vi "Read JSON from Stream.vi"(11 "Stream in":refnum<class "Stream.lvclass">) -> (0 "error out":errorcluster, 2 "Data":string)   [LabVIEW 2020, in "Stream-Simple-Msg.lvlib" / "Endpoint.lvclass"]
uses:
  Endpoint.lvclass
  <vilib>/IlluminatedG/lv-stream/stream/Stream.lvclass
  <vilib>/IlluminatedG/lv-web-crypto/lv-json/JSON/JSON Item Type.ctl
  <vilib>/IlluminatedG/lv-web-crypto/lv-json/JSON/JSON.lvlib
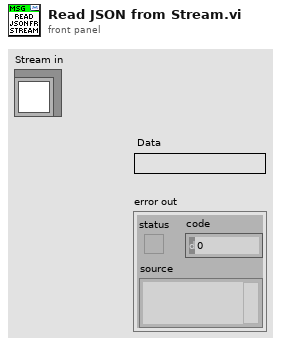
[diagram p1: front panel]
types:
  T1 = typedef "JSON.lvlib/JSON Item Type.ctl" = enum16{"unknown", "null", "Array", "Object", "String", "Number", "Boolean"}
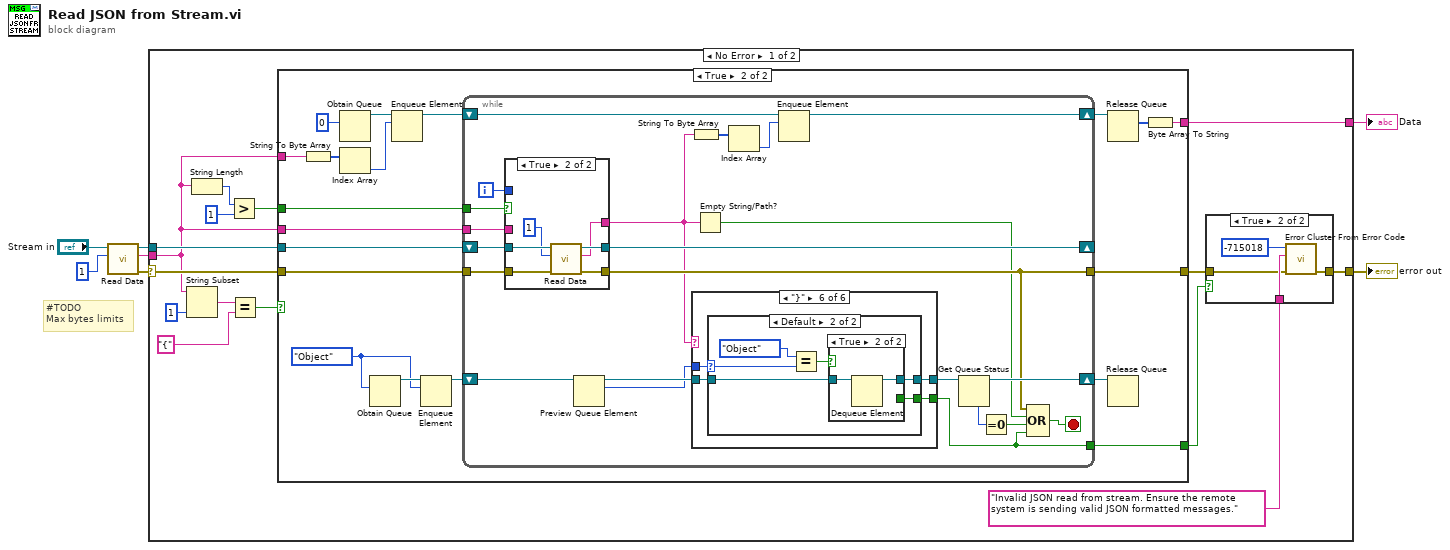
[diagram p0: block diagram]
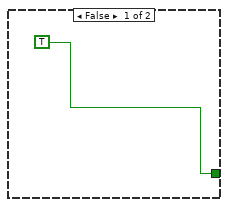
[diagram p2: hidden frame]
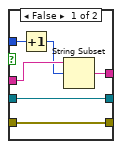
[diagram p3: hidden frame]
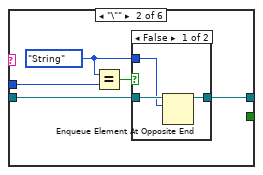
[diagram p5: hidden frame]
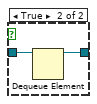
[diagram p6: hidden frame]
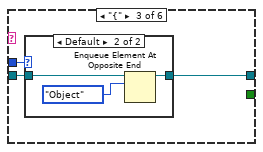
[diagram p7: hidden frame]
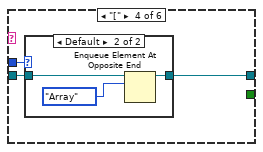
[diagram p9: hidden frame]
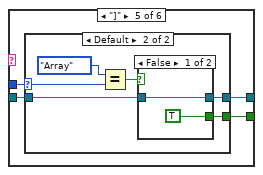
[diagram p11: hidden frame]
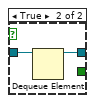
[diagram p13: hidden frame]
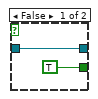
[diagram p15: hidden frame]
diagram:
  # "#TODO\nMax bytes limits"
  n1 = call <vilib>:"Read Data.vi"("Count"=1, "Stream in"="Stream in") -> ("error out"=w2:errorcluster, "Data"=w1:string, "Stream out"=w5:refnum<class "Stream.lvclass">)  [unwired: 7 in]
  n2 = case shown="No Error" w2 {
    selector: w2 -> [w14 w137]
    tunnel: w5 -> [w19 _]
    tunnel: [w18 _] -> w4
    tunnel: [w16 w137] -> w3
    tunnel: w1 -> [w11 _]
    frame No Error {
      n3 = String Subset(string=w11, length (rest)=1 ("length (rest)")) -> (substring=w12:string)  [unwired: 1 in]
      n4 = String Length(string=w11) -> (length=w10:i32)
      n5 = Greater?(x=w10, y=1) -> (0:w8:bool)
      n6 = Equal?(x=w12, y="{") -> (x = y?=w20:bool)
      n7 = case shown="True" w20 {
        tunnel: w11 -> [_ w34]
        tunnel: w19 -> [_ w39]
        tunnel: [_ w29] -> w18
        tunnel: [TRUE w28] -> w17
        tunnel: w14 -> [_ w27]
        tunnel: [_ w26] -> w22
        tunnel: w11 -> [_ w25]
        tunnel: w8 -> [_ w24]
        frame False {
        }
        frame True {
          w37 = JSON_Item_Type."Object" ("element")
          n8 = String To Byte Array(string=w34) -> (unsigned byte array=w33:u8[])
          n9 = Obtain Queue(element data type=u8 0) -> (queue out=w38:refnum<queue>)  [unwired: 4 in, 2 out]
          n10 = Index Array(array=w33) -> (element=w32:u8)  [unwired: 1 in]
          n11 = Obtain Queue(element data type=w37) -> (queue out=w42:refnum<queue>)  [unwired: 4 in, 2 out]
          n12 = Enqueue Element(queue=w38, element=w32) -> (queue out=w36:refnum<queue>)  [unwired: 2 in, 2 out]
          n13 = Enqueue Element(queue=w42, element=w37) -> (queue out=w41:refnum<queue>)  [unwired: 2 in, 2 out]
          n14 = while {
            shift-right: [w59] -> w40
            shift-left: w41 -> [w63]
            tunnel: [w51] -> w28
            shift-right: [w52] -> w31
            shift-left: w36 -> [w55]
            shift-right: [w50] -> _
            shift-left: w39 -> [w56]
            tunnel: w27 -> [w49]
            tunnel: [w45] -> w26
            tunnel: w25 -> [w46]
            tunnel: w24 -> [w48]
            i -> [w47]
            stop <- w64 stop-if-true
            n15 = case shown="True" w48 {
              tunnel: [w69 w76] -> w45
              tunnel: w56 -> [w70 w75]
              tunnel: [w67 w71] -> w44
              tunnel: [w70 w74] -> w50
              tunnel: w49 -> [w69 w73]
              tunnel: w47 -> [w66 _]
              tunnel: w46 -> [w68 _]
              frame False {
                n16 = Increment(x=w66) -> (x+1=w65:i32)
                n17 = String Subset(string=w68, offset (0)=w65) -> (substring=w67:string)  [unwired: 1 in]
              }
              frame True {
                n18 = call <vilib>:"Read Data.vi"("error in (no error)"=w73, "Count"=1, "Stream in"=w75) -> ("error out"=w76:errorcluster, "Data"=w71:string, "Stream out"=w74:refnum<class "Stream.lvclass">)  [unwired: 6 in]
              }
            }
            n19 = Preview Queue Element(queue=w63) -> (queue out=w62:refnum<queue>, element=w61:T1)  [unwired: 2 in, 2 out]
            n20 = String To Byte Array(string=w44) -> (unsigned byte array=w54:u8[])
            n21 = case shown="\"}\"" w44 {
              tunnel: w61 -> [_ w81 w88 w95 w103 w118]
              tunnel: w62 -> [w77 w80 w90 w97 w105 w120]
              tunnel: [w77 w79 w89 w96 w104 w119] -> w60
              tunnel: [_ _ _ _ w102 w117] -> w51
              frame Default {
              }
              frame "\"" {
                w78 = JSON_Item_Type."String" ("JSON Item Type")
                n22 = Equal?(x=w78, y=w81) -> (x = y?=w82:bool)
                n23 = case shown="False" w82 {
                  tunnel: w80 -> [w85 w87]
                  tunnel: [w84 w86] -> w79
                  tunnel: w78 -> [w83 _]
                  frame False {
                    n24 = Enqueue Element At Opposite End(queue=w85, element=w83) -> (queue out=w84:refnum<queue>)  [unwired: 2 in, 2 out]
                  }
                  frame True {
                    n25 = Dequeue Element(queue=w87) -> (queue out=w86:refnum<queue>)  [unwired: 2 in, 3 out]
                  }
                }
              }
              frame "{" {
                n26 = case shown="Default" w88 {
                  tunnel: w90 -> [w91 w94]
                  tunnel: [w91 w93] -> w89
                  frame "String" {
                  }
                  frame Default {
                    n27 = Enqueue Element At Opposite End(queue=w94, element=JSON_Item_Type."Object" ("JSON Item Type")) -> (queue out=w93:refnum<queue>)  [unwired: 2 in, 2 out]
                  }
                }
              }
              frame "[" {
                n28 = case shown="Default" w95 {
                  tunnel: w97 -> [w98 w101]
                  tunnel: [w98 w100] -> w96
                  frame "String" {
                  }
                  frame Default {
                    n29 = Enqueue Element At Opposite End(queue=w101, element=JSON_Item_Type."Array" ("JSON Item Type")) -> (queue out=w100:refnum<queue>)  [unwired: 2 in, 2 out]
                  }
                }
              }
              frame "]" {
                n30 = case shown="Default" w103 {
                  selector: w103 -> [_ w112]
                  tunnel: w105 -> [w106 w110]
                  tunnel: [w106 w109] -> w104
                  tunnel: [_ w108] -> w102
                  frame "String" {
                  }
                  frame Default {
                    n31 = Equal?(x=JSON_Item_Type."Array" ("JSON Item Type"), y=w112) -> (x = y?=w111:bool)
                    n32 = case shown="False" w111 {
                      tunnel: w110 -> [w114 w116]
                      tunnel: [w114 w115] -> w109
                      tunnel: [TRUE _] -> w108
                      frame False {
                      }
                      frame True {
                        n33 = Dequeue Element(queue=w116) -> (queue out=w115:refnum<queue>)  [unwired: 2 in, 3 out]
                      }
                    }
                  }
                }
              }
              frame "}" {
                n34 = case shown="Default" w118 {
                  selector: w118 -> [_ w127]
                  tunnel: w120 -> [w121 w125]
                  tunnel: [w121 w124] -> w119
                  tunnel: [_ w123] -> w117
                  frame "String" {
                  }
                  frame Default {
                    n35 = Equal?(x=JSON_Item_Type."Object" ("JSON Item Type"), y=w127) -> (x = y?=w126:bool)
                    n36 = case shown="True" w126 {
                      tunnel: w125 -> [w129 w131]
                      tunnel: [w129 w130] -> w124
                      tunnel: [TRUE _] -> w123
                      frame False {
                      }
                      frame True {
                        n37 = Dequeue Element(queue=w131) -> (queue out=w130:refnum<queue>)  [unwired: 2 in, 3 out]
                      }
                    }
                  }
                }
              }
            }
            n38 = Empty String/Path?(string/path=w44) -> (empty?=w43:bool)
            n39 = Index Array(array=w54) -> (element=w53:u8)  [unwired: 1 in]
            n40 = Enqueue Element(queue=w55, element=w53) -> (queue out=w52:refnum<queue>)  [unwired: 2 in, 2 out]
            n41 = Get Queue Status(queue=w60) -> (queue out=w59:refnum<queue>, # elements in queue=w58:i32)  [unwired: 2 in, 6 out]
            n42 = Equal To 0?(x=w58) -> (x = 0?=w57:bool)
            n43 = Compound Arithmetic op=OR(w45, w43, w57, w51) -> (w64:bool)
          }
          n44 = Release Queue(queue=w31) -> (remaining elements=w30:u8[])  [unwired: 2 in, 2 out]
          n45 = Release Queue(queue=w40) -> ()  [unwired: 2 in, 3 out]
          n46 = Byte Array To String(unsigned byte array=w30) -> (string=w29:string)
        }
      }
      n47 = case shown="True" w17 {
        tunnel: [w132 w135] -> w16
        tunnel: "Invalid JSON read from stream. Ensure the remote system is sending valid JSON formatted messages." ("error message (\"\")") -> [_ w134]
        tunnel: w22 -> [w132 w133]
        frame False {
        }
        frame True {
          n48 = call <vilib>:"Error Cluster From Error Code.vi"("error in (no error)"=w133, "error message (\"\")"=w134, "error code (0)"=-715018) -> ("error out"=w135:errorcluster)  [unwired: 6 in]
        }
      }
    }
    frame Error {
    }
  }
  "error out" <- w3
  "Data" <- w4
